vi "子VI-查看某框-只读穿透图模式.vi"(0 "输入框号（默认值0为整张图）":dbl format="%#_13g", 1 "框组":T3(array[cluster]), 2 "临界Z值":i32, 4 "临界面积百分比值":dbl, 5 "预先配置的灰度阈值":dbl, 6 "穿透图原始路径":path, 7 "部位信息":string[](array[string])=["", "34.500000", "32.500000", "1121", "34", "54.955926", "分层类", "不合格", ""], 12 "产品规格":cluster{"产品长度（周长）（mm）":dbl, "产品宽度（母线长）（mm）":dbl}) -> (14 "?":string[][](table), 19 "全部检测结果":string[][](table))   [LabVIEW 2018]
uses:
  <vilib>/vision/NI_Vision_Development_Module.lvlib
panel:
  in  "格式字符串 4":string="%f"
  in  "分隔符（'\\'代码显示） 3":string="\t"
  in  "返回主界面":bool caption="辅助定性分析"
  in  "Tab Control":T1
  out "?":T2(plugin-control)
  out "Threshold Image":T2(plugin-control)
  out "Threshold Image":T2(plugin-control)
  in  "格式字符串 3":string="%f"
  in  "分隔符（'\\'代码显示） 2":string="\t"
  out "弥散和分层临界灰度值":i64
  out "弥散缺陷个数":i32
  out "分层缺陷个数":i32
  out "合格？ 弥散类":string="fencengThreshold"
  out "合格？分层类":string="fencengThreshold"
  out "弥散测量结果":i16[][](array[numeric])
  out "弥散类检测结果":string[][](table)
  out "?":string
  out "面积 (pixels)":i32
  in  "格式字符串 2":string="%f"
  in  "分隔符（'\\'代码显示）":string="\t"
  out "分层测量结果":i16[][](array[numeric])
  out "缺陷初步分类的临界值":sgl format="%#.3f"
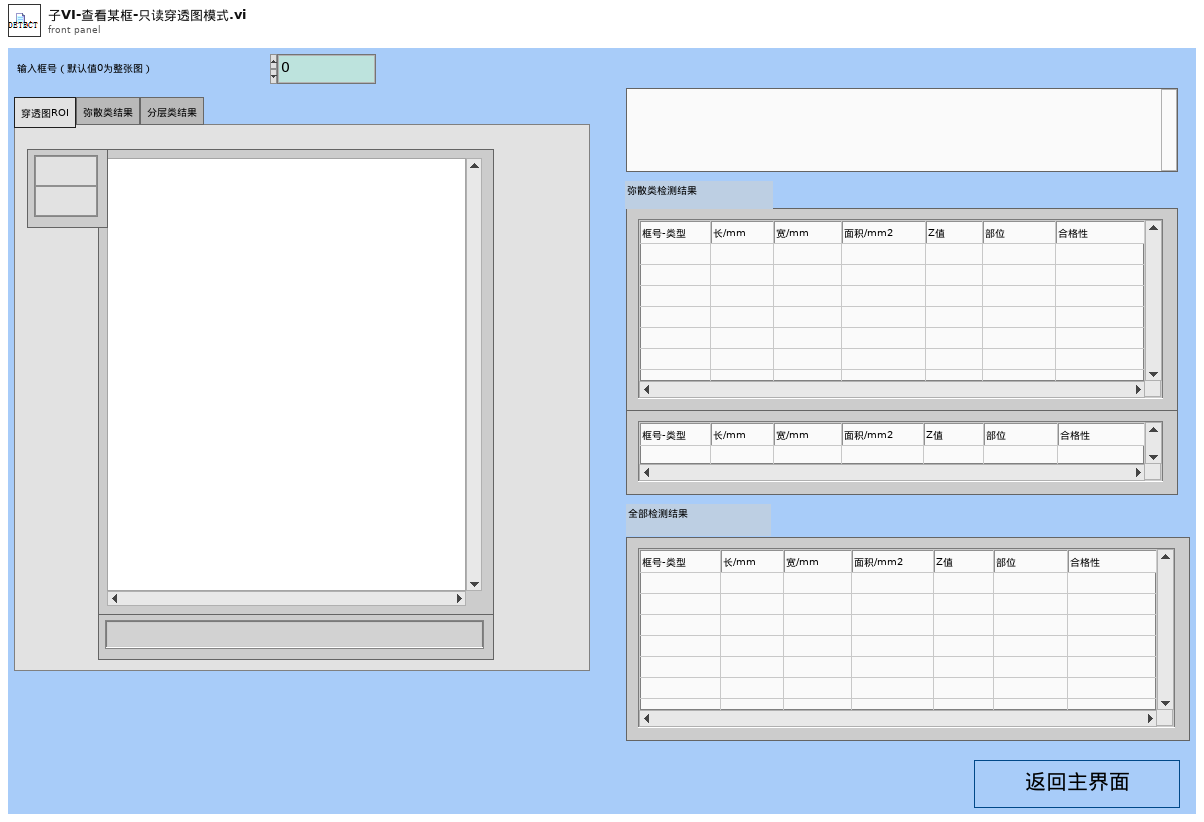
[diagram p1: front panel]
types:
  T1 = typedef "控件2.ctl" = enum32{"穿透图ROI", "弥散类结果", "分层类结果"}
  T2 = typedef "IMAQ Image.ctl" = refnum<image>
  T3 = cluster{"Global Rectangle":i32[], "Contours":cluster{"Contour Type":u32, "ROI Type":u32, "Points":i32[]}[]}[]
  T4 = cluster{"Zoom Tool":bool, "Selection Tool":bool, "Pan Tool":bool, "Point Tool":bool, "Line Tool":bool, "Rectangle Tool":bool, "Rotated Rectangle Tool":bool, "Polyline Tool":bool, "Polygon Tool":bool, "Freehand Tool":bool, "Closed Freehand Tool":bool, "Ellipse Tool":bool, "Annulus Tool":bool}
  T5 = typedef "Image Type" = u32
  T6 = cluster{"Global Rectangle":i32[], "Contours":cluster{"Contour Type":u32, "ROI Type":u32, "Points":i32[]}[]}
  T7 = typedef "Particle Parameters" = i32
  T8 = cluster{"Measurement Parameter":T7, "Range Lower Value":dbl, "Range Upper Value":dbl, "Range":bool, "Measurement Type":bool}[]
  T9 = cluster{"histogram":u32[], "Minimal Value":sgl, "Maximal Value":sgl, "Starting Value":sgl, "Interval Width":sgl, "Mean Value":sgl, "Standard  Variation":sgl, "Area (pixels)":i32}
  T10 = cluster{"Area":dbl, "Number of Holes":dbl, "Bounding Rect":cluster{"Left":dbl, "Top":dbl, "Right":dbl, "Bottom":dbl}, "Center of Mass":cluster{"X":dbl, "Y":dbl}, "Orientation":dbl, "Dimensions":cluster{"Width":dbl, "Height":dbl}}[]
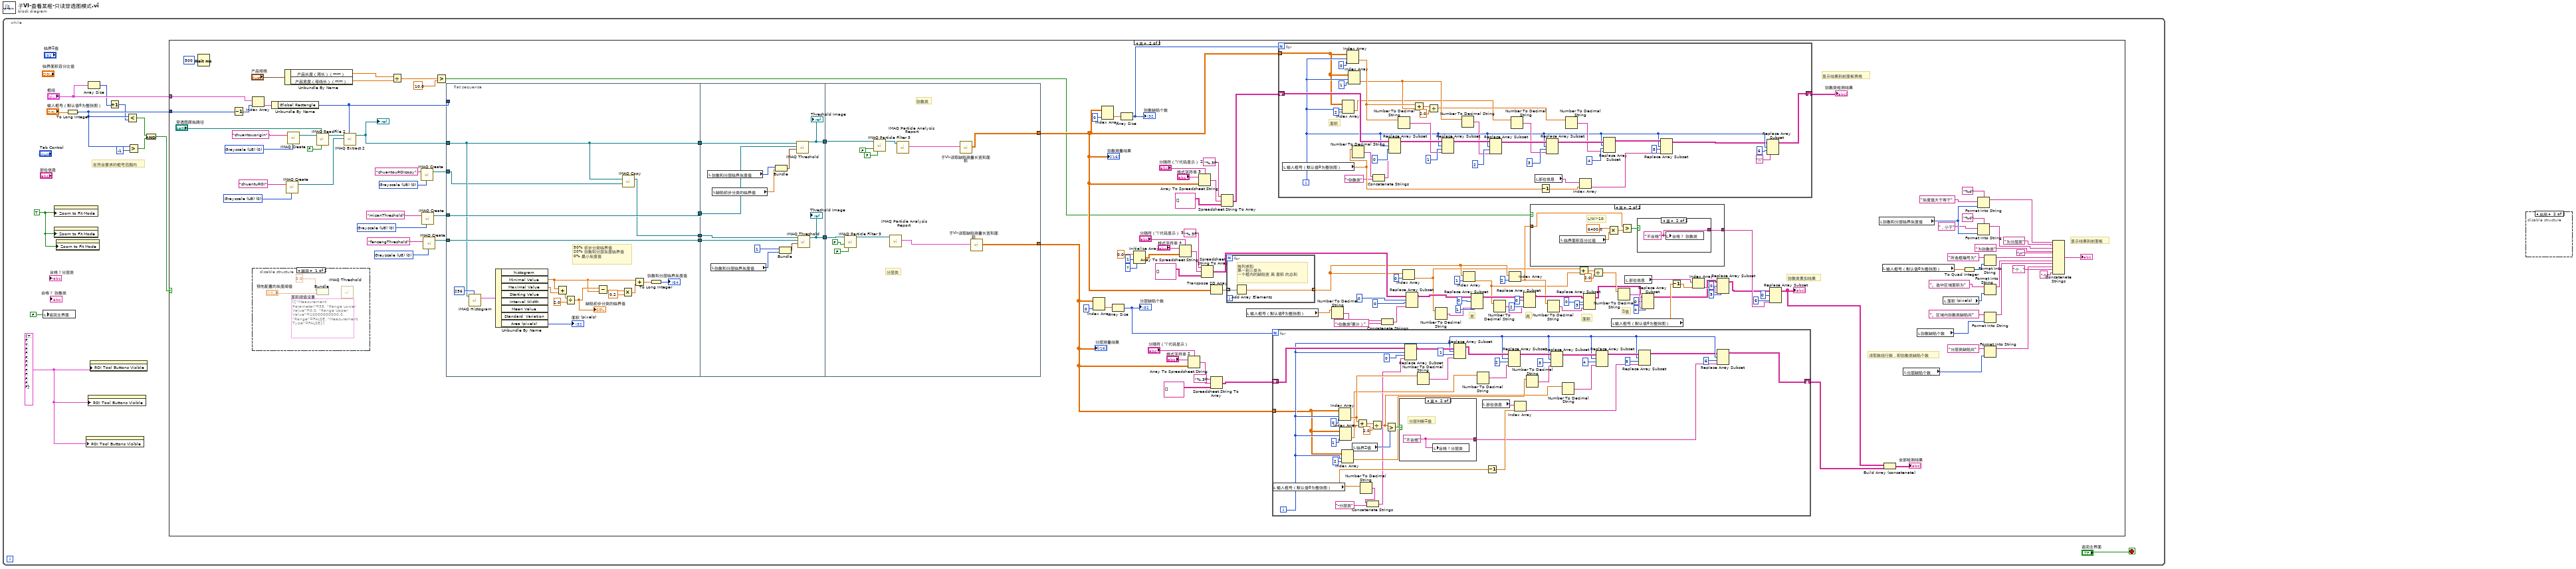
[diagram p0: block diagram]
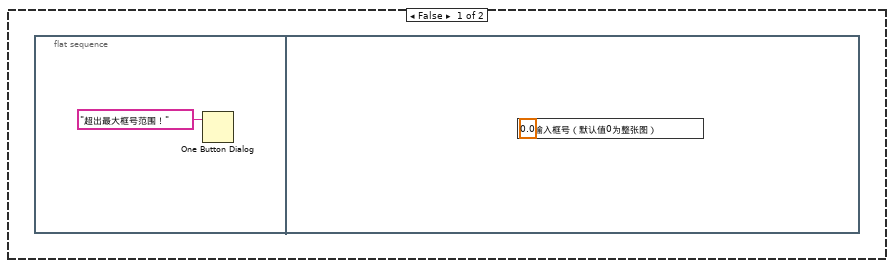
[diagram p2: hidden frame]
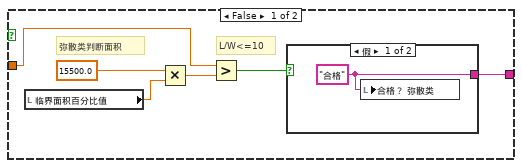
[diagram p3: hidden frame]
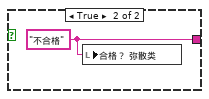
[diagram p4: hidden frame]
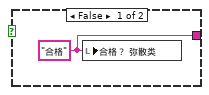
[diagram p5: hidden frame]
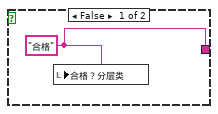
[diagram p7: hidden frame]
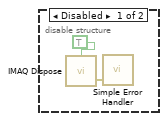
[diagram p8: hidden frame]
diagram:
  n1 = while {
    stop <- "返回主界面" stop-if-true
    w3 = T4 {"Zoom Tool"=TRUE, "Selection Tool"=FALSE, "Pan Tool"=TRUE, "Point Tool"=FALSE, "Line Tool"=FALSE, "Rectangle Tool"=FALSE, "Rotated Rectangle Tool"=FALSE, "Polyline Tool"=FALSE, "Polygon Tool"=FALSE, "Freehand Tool"=FALSE, "Closed Freehand Tool"=FALSE, "Ellipse Tool"=FALSE, "Annulus Tool"=FALSE} ("ROI Tool Buttons Visible:All Elements")
    w11 = TRUE ("Zoom to Fit Mode")
    # "在符合要求的框号范围内"
    n2 = local write "返回主界面"(FALSE ("stop")) -> ()
    n3 = property class="ImageControl"("Zoom to Fit Mode"=w11) -> ()  [unwired: 2 in, 2 out]
    n4 = property class="ImageControl"("Zoom to Fit Mode"=w11) -> ()  [unwired: 2 in, 2 out]
    n5 = property class="ImageControl"("Zoom to Fit Mode"=w11) -> ()  [unwired: 2 in, 2 out]
    n6 = To Long Integer(number="输入框号（默认值0为整张图）") -> (32bit integer=w5:i32)
    n7 = property class="ImageControl"("ROI Tool Buttons Visible"=w3) -> ()  [unwired: 2 in, 2 out]
    n8 = Array Size(array="框组") -> (size(s)=w2:i32)
    n9 = property class="ImageControl"("ROI Tool Buttons Visible"=w3) -> ()  [unwired: 2 in, 2 out]
    n10 = property class="ImageControl"("ROI Tool Buttons Visible"=w3) -> ()  [unwired: 2 in, 2 out]
    n11 = Increment(x=w2) -> (x+1=w1:i32)
    n12 = Less?(x=w5, y=w1) -> (x < y?=w7:bool)
    n13 = Greater?(x=w5, y=-1) -> (0:w6:bool)
    n14 = And(x=w7, y=w6) -> (x .and. y?=w8:bool)
    n15 = case shown="真" w8 {
      tunnel: "框组" -> [_ w80]
      tunnel: w5 -> [_ w79]
      frame False {
        n16 = flat-sequence {
          frame #0 {
            n17 = One Button Dialog(message="超出最大框号范围！" ("消息")) -> ()  [unwired: 1 in, 1 out]
          }
          frame #1 {
            n18 = local write "输入框号（默认值0为整张图）"(0.0 ("框号")) -> ()
          }
        }
      }
      frame True {
        w107 = T5 0 items=["Grayscale (U8)", "Grayscale (I16)", "Grayscale (SGL)", "Complex (CSG)", "RGB (U32)", "HSL (U32)", "RGB (U64)", "Grayscale (U16)"] ("Image Type")
        w130 = T5 0 items=["Grayscale (U8)", "Grayscale (I16)", "Grayscale (SGL)", "Complex (CSG)", "RGB (U32)", "HSL (U32)", "RGB (U64)", "Grayscale (U16)"] ("Image Type")
        w131 = T5 0 items=["Grayscale (U8)", "Grayscale (I16)", "Grayscale (SGL)", "Complex (CSG)", "RGB (U32)", "HSL (U32)", "RGB (U64)", "Grayscale (U16)"] ("Image Type")
        w134 = T5 0 items=["Grayscale (U8)", "Grayscale (I16)", "Grayscale (SGL)", "Complex (CSG)", "RGB (U32)", "HSL (U32)", "RGB (U64)", "Grayscale (U16)"] ("Image Type")
        w147 = T5 0 items=["Grayscale (U8)", "Grayscale (I16)", "Grayscale (SGL)", "Complex (CSG)", "RGB (U32)", "HSL (U32)", "RGB (U64)", "Grayscale (U16)"] ("Image Type")
        # "Z值"
        # "面积"
        # "高"
        # "宽"
        # "弥散类累加结果"
        # "显示结果到前面板"
        # "读取数组行数，即弥散类缺陷个数"
        # "显示结果到前面板表格"
        n19 = Wait (ms)(milliseconds to wait=u32 500 ("等待时间（毫秒）")) -> ()  [unwired: 1 out]
        n20 = Decrement(x=w79) -> (x-1=w149:i32)
        n21 = Index Array(array=w80, index=w149) -> (element=w150:T6)
        n22 = disable-structure shown="禁用" {
          frame Disabled {
            (unwired) T8 [{"Measurement Parameter"=35, "Range Lower Value"=0.0, "Range Upper Value"=10000000000.0, "Range"=FALSE, "Measurement Type"=FALSE}]  # 面积阈值设置
            n23 = Bundle(0.0, "预先配置的灰度阈值"="预先配置的灰度阈值") -> ()  [unwired: 1 in, 1 out]
            n24 = call "IMAQ Threshold"() -> ()  [unwired: 6 in, 6 out]
          }
          frame Enabled {
          }
        }
        n25 = Unbundle By Name(w150) -> ("Global Rectangle"=w125:i32[])
        n26 = Unbundle By Name("产品规格") -> ("产品长度（周长）（mm）"=w141:dbl, "产品宽度（母线长）（mm）"=w140:dbl)
        n27 = call "IMAQ Create"("Image Name"="chuantuROI", "Image Type"=w134) -> ("New Image"=w133:T2)  [unwired: 3 in, 1 out]
        n28 = call "IMAQ Create"("Image Name"="chuantouorigin", "Image Type"=w147) -> ("New Image"=w136:T2)  [unwired: 3 in, 1 out]
        n29 = call "IMAQ ReadFile 2"("Use File Path Image Type"=FALSE, "File Path"="穿透图原始路径", "Image"=w136) -> ("Image Out"=w137:T2)  [unwired: 4 in, 4 out]
        n30 = call "IMAQ Extract 2"("Optional Rectangle"=w125, "Image Dst"=w133, "Image Src"=w137) -> ("Image Dst Out"=w110:T2)  [unwired: 7 in, 1 out]
        "?" <- w110
        n31 = Divide(x=w141, y=w140) -> (x/y=w144:dbl)
        n32 = call "IMAQ Create"("Image Name"="chuantouROIcopy", "Image Type"=w107) -> ("New Image"=w109:T2)  [unwired: 3 in, 1 out]
        n33 = call "IMAQ Create"("Image Name"="misanThreshold", "Image Type"=w130) -> ("New Image"=w124:T2)  [unwired: 3 in, 1 out]
        n34 = call "IMAQ Create"("Image Name"="fencengThreshold", "Image Type"=w131) -> ("New Image"=w123:T2)  [unwired: 3 in, 1 out]
        n35 = Greater?(x=w144, y=10.0) -> (0:w30:bool)
        n36 = flat-sequence {
          tunnel: [w236] -> w156
          tunnel: [w235] -> w155
          tunnel: [w221] -> w154
          tunnel: [w220] -> w153
          tunnel: w125 -> [_]
          tunnel: w124 -> [w236]
          tunnel: w123 -> [w235]
          tunnel: w110 -> [w221]
          tunnel: w109 -> [w219]
          tunnel: w156 -> [w248]
          tunnel: w155 -> [w247]
          tunnel: [w237] -> w152
          tunnel: [w240] -> w151
          tunnel: w154 -> [w241]
          tunnel: w153 -> [w239]
          tunnel: [w249] -> w74
          tunnel: w152 -> [w256]
          tunnel: w151 -> [w255]
          tunnel: [w252] -> w77
          frame #0 {
            # "50% 初步分类临界值\n20% 弥散和分层灰度临界值\n0% 最小灰度值"
            n37 = call "IMAQ Histogram"("Number of Classes"=256, "Image"=w221) -> ("Histogram Report"=w233:T9)  [unwired: 8 in, 1 out]
            n38 = Unbundle By Name(w233) -> ("Minimal Value"=w223:sgl, "Maximal Value"=w229:sgl, "Area (pixels)"=→"面积 (pixels)":i32)  [unwired: 5 out]
            n39 = Add(x=w223, y=w229) -> (x+y=w228:sgl)
            n40 = Divide(x=w228, y=sgl 2.0) -> (x/y=w227:sgl)
            "缺陷初步分类的临界值" <- w227
            n41 = Subtract(x=w227, y=w223) -> (x-y=w225:sgl)
            n42 = Multiply(x=w225, y=0.2) -> (x*y=w224:dbl)
            n43 = call "IMAQ Copy"("Image Dst"=w219, "Image Src"=w221) -> ("Image Dst Out"=w220:T2)  [unwired: 4 in, 1 out]
            n44 = Add(x=w223, y=w224) -> (x+y=w222:dbl)
            n45 = To Long Integer(number=w222) -> (32bit integer=→"弥散和分层临界灰度值":i32)
          }
          frame #1 {
            n46 = local read "弥散和分层临界灰度值"() -> (w238:i64)
            n47 = local read "弥散和分层临界灰度值"() -> (w243:i64)
            n48 = local read "缺陷初步分类的临界值"() -> (w245:sgl)
            n49 = Bundle("弥散和分层临界灰度值"=w238, "缺陷初步分类的临界值"=w245) -> (w246:cluster{"弥散和分层临界灰度值":i64, "缺陷初步分类的临界值":sgl})  [unwired: 1 in]
            n50 = Bundle(1, "弥散和分层临界灰度值"=w243) -> (w242:cluster{i32, "弥散和分层临界灰度值":i64})  [unwired: 1 in]
            n51 = call "IMAQ Threshold"("Range"=w246, "Image Dst"=w248, "Image Src"=w241) -> ("Image Dst Out"=w240:T2)  [unwired: 3 in, 5 out]
            "Threshold Image" <- w240
            n52 = call "IMAQ Threshold"("Range"=w242, "Image Dst"=w247, "Image Src"=w239) -> ("Image Dst Out"=w237:T2)  [unwired: 3 in, 5 out]
            "Threshold Image" <- w237
          }
          frame #2 {
            # "分层类"
            # "弥散类"
            n53 = call "IMAQ Particle Filter 3"("Image Src"=w256, "Keep/Remove Particles (F)"=FALSE, "Reject Border? (F)"=FALSE) -> ("Image Dst Out"=w254:T2)  [unwired: 10 in, 2 out]
            n54 = call "IMAQ Particle Filter 3"("Image Src"=w255, "Keep/Remove Particles (F)"=FALSE, "Reject Border? (F)"=FALSE) -> ("Image Dst Out"=w251:T2)  [unwired: 10 in, 2 out]
            n55 = call "IMAQ Particle Analysis Report"("Image"=w254) -> ("Particle Reports (Pixels)"=w253:T10)  [unwired: 5 in, 5 out]
            n56 = call "IMAQ Particle Analysis Report"("Image"=w251) -> ("Particle Reports (Pixels)"=w250:T10)  [unwired: 5 in, 5 out]
            n57 = call "子VI-读取缺陷测量长宽和面积.vi"("Particle Reports (Pixels)"=w250) -> ("测量结果"=w249:dbl[][])  [unwired: 10 in]
            n58 = call "子VI-读取缺陷测量长宽和面积.vi"("Particle Reports (Pixels)"=w253) -> ("测量结果"=w252:dbl[][])  [unwired: 10 in]
          }
        }
        n59 = Index Array(array=w77, index (col)=0 ("禁用的索引 (列)")) -> (element=w129:dbl[])  [unwired: 1 in]
        n60 = Index Array(array=w74, index (col)=0 ("禁用的索引 (列)")) -> (element=w127:dbl[])  [unwired: 1 in]
        n61 = Array Size(array=w129) -> (size(s)=w122:i32)
        "分层缺陷个数" <- w122
        n62 = Array Size(array=w127) -> (size(s)=w139:i32)
        "弥散缺陷个数" <- w139
        n63 = Initialize Array(0.0 ("元素"), 1 ("维数大小"), 7 ("维数大小")) -> (w62:dbl[][])
        n64 = Array To Spreadsheet String(delimiter (Tab)="分隔符（'\\'代码显示） 3", array=w62, 3:"格式字符串 4") -> (spreadsheet string=w65:string)
        n65 = Array To Spreadsheet String(delimiter (Tab)="分隔符（'\\'代码显示）", array=w77, 3:"格式字符串 2") -> (spreadsheet string=w119:string)
        n66 = Array To Spreadsheet String(delimiter (Tab)="分隔符（'\\'代码显示） 2", array=w74, 3:"格式字符串 3") -> (spreadsheet string=w114:string)
        n67 = Spreadsheet String To Array(format string="%.3f", spreadsheet string=w65, array type (2D Dbl)=string[][] [] ("Array")) -> (array=w61:string[][])  [unwired: 1 in]
        n68 = Transpose 2D Array(2D array=w74) -> (transposed array=w75:dbl[][])
        n69 = Spreadsheet String To Array(format string="%.3f" ("格式字符串"), spreadsheet string=w119, array type (2D Dbl)=string[][] [] ("Array")) -> (array=w117:string[][])  [unwired: 1 in]
        n70 = Spreadsheet String To Array(format string="%.3f", spreadsheet string=w114, array type (2D Dbl)=string[][] [] ("Array")) -> (array=w73:string[][])  [unwired: 1 in]
        n71 = for {
          tunnel: w75 -> [w174] mode=indexing
          tunnel: [w173] -> w47 mode=indexing
          # "按列求和 \n第一到三类为\n一个框内的缺陷宽 高 面积 的总和"
          n72 = Add Array Elements(numeric array=w174) -> (sum=w173:dbl)
        }
        n73 = local read "输入框号（默认值0为整张图）"() -> (w23:dbl)
        n74 = for {
          N: w122 -> [_]
          tunnel: w77 -> [w182]
          shift-right: [w191] -> w17
          shift-left: w117 -> [w200]
          i -> [w183]
          n75 = local read "输入框号（默认值0为整张图）"() -> (w207:dbl)
          n76 = Index Array(array=w182, index (row)=w183, index (col)=0 ("禁用的索引 (列)")) -> (element=w190:dbl)
          n77 = Index Array(array=w182, index (row)=w183, index (col)=1 ("禁用的索引 (列)")) -> (element=w189:dbl)
          n78 = Index Array(array=w182, index (row)=w183, index (col)=2 ("索引 (列)")) -> (element=w181:dbl)
          n79 = local read "临界Z值"() -> (w214:i32)
          n80 = Add(x=w190, y=w189) -> (x+y=w215:dbl)
          n81 = Number To Decimal String(number=w207) -> (decimal integer string=w179:string)  [unwired: 1 in]
          n82 = Concatenate Strings(w179, "-分层类" ("新元素/子数组")) -> (w178:string)
          n83 = Divide(x=w215, y=2.0) -> (x/y=w187:dbl)
          n84 = Greater?(x=w187, y=w214) -> (0:w216:bool)
          n85 = case shown="真" w216 {
            tunnel: [w217 w218] -> w185
            frame False {
              w217 = "合格" ("合格？")
              n86 = local write "合格？分层类"(w217) -> ()
            }
            frame True {
              w218 = "不合格" ("合格？")
              # "分层判断Z值"
              n87 = local write "合格？分层类"(w218) -> ()
            }
          }
          n88 = Replace Array Subset(array=w200, new element=w178, index (row)=w183, index (col)=0 ("索引 (列)")) -> (w199:string[][])
          n89 = Number To Decimal String(number=w190) -> (decimal integer string=w198:string)  [unwired: 1 in]
          n90 = Replace Array Subset(array=w199, new element=w198, index (row)=w183, index (col)=1 ("索引 (列)")) -> (w196:string[][])
          n91 = Number To Decimal String(number=w189) -> (decimal integer string=w197:string)  [unwired: 1 in]
          n92 = local read "部位信息"() -> (w210:string[])
          n93 = Decrement(x=w207) -> (x-1=w209:dbl)
          n94 = Replace Array Subset(array=w196, new element=w197, index (row)=w183, index (col)=2 ("索引 (列)")) -> (w195:string[][])
          n95 = Index Array(array=w210, index=w209) -> (element=w186:string)
          n96 = Number To Decimal String(number=w181) -> (decimal integer string=w194:string)  [unwired: 1 in]
          n97 = Replace Array Subset(array=w195, new element=w194, index (row)=w183, index (col)=3 ("索引 (列)")) -> (w193:string[][])
          n98 = Number To Decimal String(number=w187) -> (decimal integer string=w188:string)  [unwired: 1 in]
          n99 = Replace Array Subset(array=w193, new element=w188, index (row)=w183, index (col)=4 ("索引 (列)")) -> (w192:string[][])
          n100 = Replace Array Subset(array=w192, new element=w186, index (row)=w183, index (col)=5 ("索引 (列)")) -> (w177:string[][])
          n101 = Replace Array Subset(array=w177, new element=w185, index (row)=w183, index (col)=6 ("索引 (列)")) -> (w191:string[][])
        }
        n102 = for {
          N: w139 -> [_]
          tunnel: w74 -> [w267]
          shift-right: [w283] -> w111
          shift-left: w73 -> [w289]
          i -> [w269]
          # "面积"
          n103 = local read "输入框号（默认值0为整张图）"() -> (w271:dbl)
          n104 = Index Array(array=w267, index (row)=w269, index (col)=2 ("索引 (列)")) -> (element=w266:dbl)
          n105 = Index Array(array=w267, index (row)=w269, index (col)=0 ("禁用的索引 (列)")) -> (element=w277:dbl)
          n106 = Index Array(array=w267, index (row)=w269, index (col)=1 ("禁用的索引 (列)")) -> (element=w276:dbl)
          n107 = Number To Decimal String(number=w271) -> (decimal integer string=w263:string)  [unwired: 1 in]
          n108 = Concatenate Strings(w263, "-弥散类" ("新元素/子数组")) -> (w262:string)
          n109 = Replace Array Subset(array=w289, new element=w262, index (row)=w269, index (col)=0 ("索引 (列)")) -> (w288:string[][])
          n110 = Number To Decimal String(number=w277) -> (decimal integer string=w282:string)  [unwired: 1 in]
          n111 = Add(x=w277, y=w276) -> (x+y=w279:dbl)
          n112 = Divide(x=w279, y=2.0) -> (x/y=w275:dbl)
          n113 = Replace Array Subset(array=w288, new element=w282, index (row)=w269, index (col)=1 ("索引 (列)")) -> (w287:string[][])
          n114 = Number To Decimal String(number=w276) -> (decimal integer string=w281:string)  [unwired: 1 in]
          n115 = Replace Array Subset(array=w287, new element=w281, index (row)=w269, index (col)=2 ("索引 (列)")) -> (w286:string[][])
          n116 = Number To Decimal String(number=w266) -> (decimal integer string=w280:string)  [unwired: 1 in]
          n117 = local read "部位信息"() -> (w273:string[])
          n118 = Decrement(x=w271) -> (x-1=w272:dbl)
          n119 = Replace Array Subset(array=w286, new element=w280, index (row)=w269, index (col)=3 ("索引 (列)")) -> (w285:string[][])
          n120 = Number To Decimal String(number=w275) -> (decimal integer string=w274:string)  [unwired: 1 in]
          n121 = Index Array(array=w273, index=w272) -> (element=w270:string)
          n122 = Replace Array Subset(array=w285, new element=w274, index (row)=w269, index (col)=4 ("索引 (列)")) -> (w284:string[][])
          n123 = Replace Array Subset(array=w284, new element=w270, index (row)=w269, index (col)=5 ("索引 (列)")) -> (w261:string[][])
          n124 = Replace Array Subset(array=w261, new element="\\" ("新元素/子数组"), index (row)=w269, index (col)=6 ("索引 (列)")) -> (w283:string[][])
        }
        "弥散类检测结果" <- w111
        n125 = Number To Decimal String(number=w23) -> (decimal integer string=w22:string)  [unwired: 1 in]
        n126 = Concatenate Strings(w22, "-弥散类(累计）" ("新元素/子数组")) -> (w20:string)
        n127 = Index Array(array=w47, index=0 ("索引")) -> (element=w25:dbl)
        n128 = Replace Array Subset(array=w61, new element=w20, index (row)=0 ("禁用的索引 (行)"), index (col)=0 ("索引 (列)")) -> (w57:string[][])
        n129 = Number To Decimal String(number=w25) -> (decimal integer string=w56:string)  [unwired: 1 in]
        n130 = Index Array(array=w47, index=1 ("索引")) -> (element=w24:dbl)
        n131 = Replace Array Subset(array=w57, new element=w56, index (row)=0 ("索引 (行)"), index (col)=1 ("索引 (列)")) -> (w54:string[][])
        n132 = Number To Decimal String(number=w24) -> (decimal integer string=w46:string)  [unwired: 1 in]
        n133 = Index Array(array=w47, index=2 ("索引")) -> (element=w26:dbl)
        n134 = Replace Array Subset(array=w54, new element=w46, index (row)=0 ("索引 (行)"), index (col)=2 ("禁用的索引 (列)")) -> (w49:string[][])
        n135 = case shown="真" w30 {
          tunnel: [w161 w169] -> w27
          tunnel: w26 -> [w157 w165]
          frame False {
            # "弥散类判断面积"
            # "L/W<=10"
            n136 = local read "临界面积百分比值"() -> (w159:dbl)
            n137 = Multiply(x=15500.0, y=w159) -> (x*y=w158:dbl)
            n138 = Greater?(x=w157, y=w158) -> (0:w162:bool)
            n139 = case shown="假" w162 {
              tunnel: [w163 w164] -> w161
              frame False {
                w163 = "合格" ("合格？")
                n140 = local write "合格？ 弥散类"(w163) -> ()
              }
              frame True {
                w164 = "不合格" ("合格？")
                n141 = local write "合格？ 弥散类"(w164) -> ()
              }
            }
          }
          frame True {
            # "L/W>10"
            n142 = local read "临界面积百分比值"() -> (w166:dbl)
            n143 = Multiply(x=6400.0, y=w166) -> (x*y=w168:dbl)
            n144 = Greater?(x=w165, y=w168) -> (0:w170:bool)
            n145 = case shown="真" w170 {
              tunnel: [w171 w172] -> w169
              frame False {
                w171 = "合格" ("合格？")
                n146 = local write "合格？ 弥散类"(w171) -> ()
              }
              frame True {
                w172 = "不合格" ("合格？")
                n147 = local write "合格？ 弥散类"(w172) -> ()
              }
            }
          }
        }
        n148 = Number To Decimal String(number=w26) -> (decimal integer string=w45:string)  [unwired: 1 in]
        n149 = Add(x=w25, y=w24) -> (x+y=w44:dbl)
        n150 = Replace Array Subset(array=w49, new element=w45, index (row)=0 ("索引 (行)"), index (col)=3 ("索引 (列)")) -> (w38:string[][])
        n151 = Divide(x=w44, y=2.0) -> (x/y=w42:dbl)
        n152 = local read "输入框号（默认值0为整张图）"() -> (w37:dbl)
        n153 = Number To Decimal String(number=w42) -> (decimal integer string=w41:string)  [unwired: 1 in]
        n154 = local read "部位信息"() -> (w35:string[])
        n155 = Replace Array Subset(array=w38, new element=w41, index (row)=0 ("索引 (行)"), index (col)=4 ("索引 (列)")) -> (w31:string[][])
        n156 = Decrement(x=w37) -> (x-1=w36:dbl)
        n157 = Index Array(array=w35, index=w36) -> (element=w34:string)
        n158 = Replace Array Subset(array=w31, new element=w34, index (row)=0 ("索引 (行)"), index (col)=5 ("索引 (列)")) -> (w19:string[][])
        n159 = Replace Array Subset(array=w19, new element=w27, index (row)=0 ("索引 (行)"), index (col)=6 ("索引 (列)")) -> (w18:string[][])
        "?" <- w18
        n160 = local read "弥散和分层临界灰度值"() -> (w106:i64)
        n161 = local read "输入框号（默认值0为整张图）"() -> (w97:dbl)
        n162 = Build Array (concatenate)(w18, w17) -> (→"全部检测结果":string[][])
        n163 = local read "分层缺陷个数"() -> (w82:i32)
        n164 = local read "弥散缺陷个数"() -> (w81:i32)
        n165 = local read "面积 (pixels)"() -> (w100:i32)
        n166 = To Quad Integer(1:w97) -> (0:w98:i64)
        n167 = Format Into String(format string="%d" ("格式字符串"), initial string="灰度值大于等于" ("初始字符串"), w106) -> (resulting string=w102:string)  [unwired: 1 in, 1 out]
        n168 = Format Into String(format string="%d" ("格式字符串"), initial string="，小于" ("初始字符串"), w106) -> (resulting string=w101:string)  [unwired: 1 in, 1 out]
        n169 = Format Into String(initial string="所选框编号为" ("初始字符串"), w98) -> (resulting string=w96:string)  [unwired: 2 in, 1 out]
        n170 = Format Into String(initial string="。选中区域面积为" ("字符串"), w100) -> (resulting string=w103:string)  [unwired: 2 in, 1 out]
        n171 = Format Into String(initial string="。区域内弥散类缺陷共" ("初始字符串"), w81) -> (resulting string=w104:string)  [unwired: 2 in, 1 out]
        n172 = Format Into String(initial string="分层类缺陷共" ("初始字符串"), w82) -> (resulting string=w105:string)  [unwired: 2 in, 1 out]
        n173 = Concatenate Strings(w102, "为分层类" ("初始字符串"), w101, "为弥散类" ("初始字符串"), "\n", w96, w103, w104, "个，" ("字符串"), w105, "个" ("字符串")) -> (→"?":string)
        "分层测量结果" <- w77
        "弥散测量结果" <- w74
      }
    }
  }
  n174 = disable-structure shown="启用" {
    frame Disabled {
      n175 = call "IMAQ Dispose"("All Images? (No)"=TRUE) -> ("error out"=w300:errorcluster)  [unwired: 5 in]
      n176 = call <vilib>:"Simple Error Handler.vi"("error in (no error)"=w300) -> ()  [unwired: 4 in, 5 out]
    }
    frame Enabled {
    }
  }
